vi "read_timing_array.vi"(8 "error in":errorcluster, 11 "VISA resource in":refnum<visa-resource-name>) -> (0 "error out 2":errorcluster, 3 "VISA resource out":refnum<visa-resource-name>, 4 "delay duration":dbl, 5 "duration":dbl[](array[numeric]), 7 "start time":dbl[](array[numeric]))   [LabVIEW 2011]
doc: "Reads all delay values stored in the DG645 and returns them in an array, from t0 to H.\nSee DG645 documentation for mor info."
panel:
  in  "bytes to read":u32=256
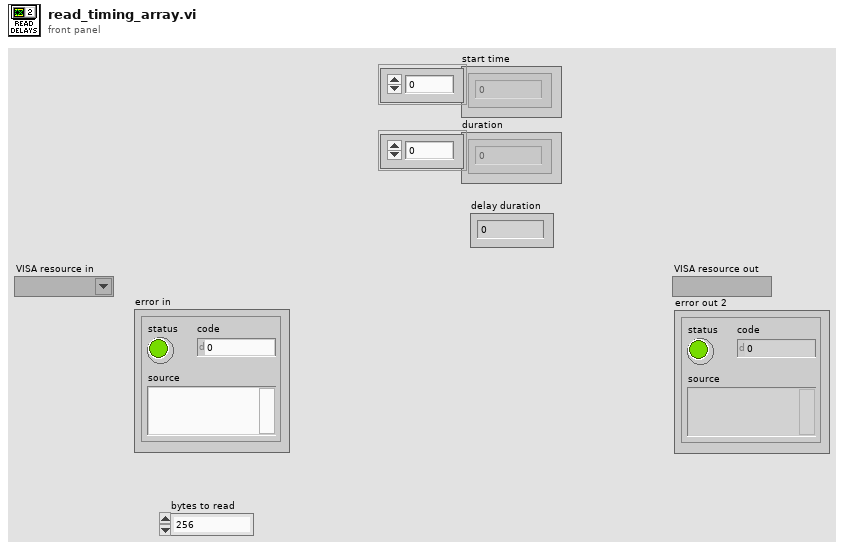
[diagram p1: front panel]
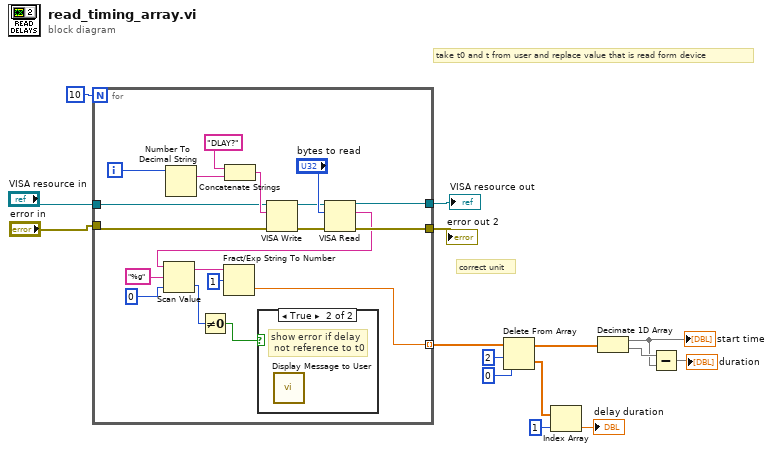
[diagram p0: block diagram]
diagram:
  # "correct unit"
  # "take t0 and t from user and replace value that is read form device"
  n1 = for {
    N: 10 -> [_]
    tunnel: "error in" -> [w31]
    tunnel: [w28] -> w7 mode=indexing
    tunnel: [w25] -> w11
    tunnel: "VISA resource in" -> [w20]
    tunnel: [w19] -> w12
    i -> [w16]
    n2 = Number To Decimal String(number=w16) -> (decimal integer string=w27:string)  [unwired: 1 in]
    n3 = Concatenate Strings("DLAY?" ("string"), w27) -> (w26:string)
    n4 = VISA Write(VISA resource name=w20, write buffer=w26, error in (no error)=w31) -> (VISA resource name out=w33:refnum<visa-resource-name>, error out=w32:errorcluster)  [unwired: 1 out]
    n5 = VISA Read(VISA resource name=w33, byte count="bytes to read", error in (no error)=w32) -> (VISA resource name out=w19:refnum<visa-resource-name>, read buffer=w18:string, error out=w25:errorcluster)  [unwired: 1 out]
    n6 = Scan Value(string=w18, format string="%g", default (0 dbl)=u16 0) -> (output string=w22:string, value=w21:u16)
    n7 = Not Equal To 0?(x=w21) -> (x != 0?=w17:bool)
    n8 = Fract/Exp String To Number(string=w22, offset=1) -> (number=w28:dbl)  [unwired: 2 in, 1 out]
    n9 = case shown="True" w17 {
      frame False {
      }
      frame True {
        # "show error if delay\n not reference to t0"
        n10 = call "Display Message to User"() -> ()  [unwired: 10 in, 2 out]
      }
    }
  }
  "VISA resource out" <- w12
  "error out 2" <- w11
  n11 = Delete From Array(array=w7, length=2, index=0) -> (deleted portion=w4:dbl[], array with subset deleted=w1:dbl[])
  n12 = Index Array(array=w4, index=1) -> (element=→"delay duration":dbl)
  n13 = Decimate 1D Array(w1) -> (w9:dbl[], w10:dbl[])
  "start time" <- w9
  n14 = Subtract(x=w10, y=w9) -> (x-y=→"duration":dbl[])
